vi "BRig_dataCurrent_Cue2Switch_Audio.vi"() -> (2 "output_Cue2Switch_Audio":i32)   [LabVIEW 2014]
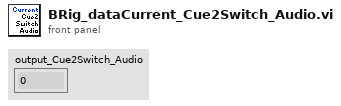
[diagram p1: front panel]
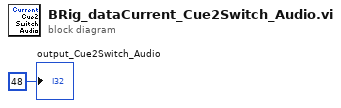
[diagram p0: block diagram]
diagram:
  "output_Cue2Switch_Audio" <- 48 ("output_iBlock")
